vi "One 8-bit Port Digital Input.vi"(2 "8-Bit DI Port":refnum<k21>="Chassis1/Mod4/DI7:0") -> (7 "Packet":u64)   [LabVIEW 2010]
uses:
  <vilib>/eio/EIONode/EIONode.xnode
  <vilib>/rvi/eio/nirviEIOImplementation/nirviEIOImplementation.xnode
  <vilib>/rvi/eio/common/nirviEmuClasses.ctl
  <vilib>/rvi/eio/common/nirviEmuTemplateMethod_noerrors.vi
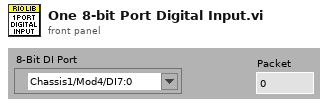
[diagram p1: front panel]
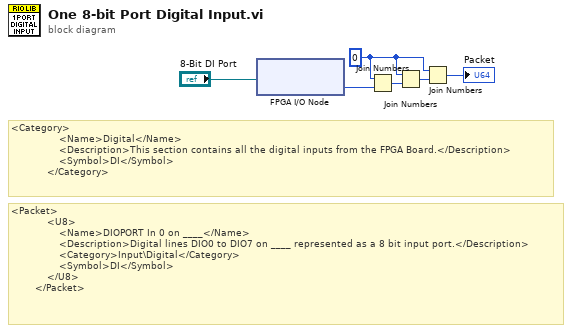
[diagram p0: block diagram]
diagram:
  w3 = u8 0 ("hi")
  # "<Packet>\n            <U8>\n                <Name>DIOPORT In 0 on ____</Name>\n                <Description>Digital lines DIO0 to DIO7 on ____ represented as a 8 bit input port.</Description>\n                <Category>Input\\Digital</Category>\n                <Symbol>DI</Symbol>\n            </U8>\n        </Packet>"
  # "<Category>\n                <Name>Digital</Name>\n                <Description>This section contains all the digital inputs from the FPGA Board.</Description>\n                <Symbol>DI</Symbol>\n            </Category>"
  n1 = xnode "FPGA I/O Node"("FPGA I/O In"="8-Bit DI Port") -> ("I/O Item"=w2:u8)  [unwired: 1 out]
  n2 = Join Numbers(hi=w3, lo=w2) -> ((hi.lo)=w5:u16)
  n3 = Join Numbers(hi=w3, lo=w5) -> ((hi.lo)=w4:u32)
  n4 = Join Numbers(hi=w3, lo=w4) -> ((hi.lo)=→"Packet":u64)
